vi "InitializeAll.vi"(8 "Error In":errorcluster) -> (0 "Error Out":errorcluster, 3 "CommunicationRefs":T8)   [LabVIEW 2015]
uses:
  TypeDefs/CoriFlowSettings.ctl
  TypeDefs/CommunicationRefs.ctl
  TypeDefs/MessageCluster.ctl
  TypeDefs/MPXSettings.ctl
  TypeDefs/ClsSettings.ctl
  TypeDefs/PDCSettings.ctl
  TypeDefs/JW24F14Settings.ctl
  TypeDefs/DAQmxAcqSettings.ctl
panel:
  in  "READY":bool
  in  "Settings":T1(tab)=enum."Photron PDC"
  in  "DAQmxAcq Settings":T2={"DAQmx Channel"="", "Simulate"=TRUE}
  in  "CoriFlowSettings":T3={"FlowBUS COM-Port"="COM3", "Node"=3, "Baud Rate"=38400, "Control Mode (0: BUS/RS232)"=enum."BUS/RS232", "Simulate"=TRUE}
  in  "ClsSettings":T4={"Connection Info (IP)"="IP: 192.168.170.2", "Simulate"=TRUE, "Load Config?"=TRUE, "Path of CLS Config"=path "C:/ADP-SLA/Drop Impact Teststand/Config/CLS.xml", "Command "=""}
  in  "MPXSettings":T5={"MPX Port"="COM4", "Simulate"=TRUE}
  in  "PDCSettings":T6={"Interface"=enum."Gigabit-Ethernet", "AutoSearch"=TRUE, "IP - AutoSearch"=[192, 168, 0], "IP - Direct"=[192, 168, 0, 9], "Simulate"=TRUE}
  in  "JW24F14Settings":T7={"Simulate"=TRUE, "device index"=0}
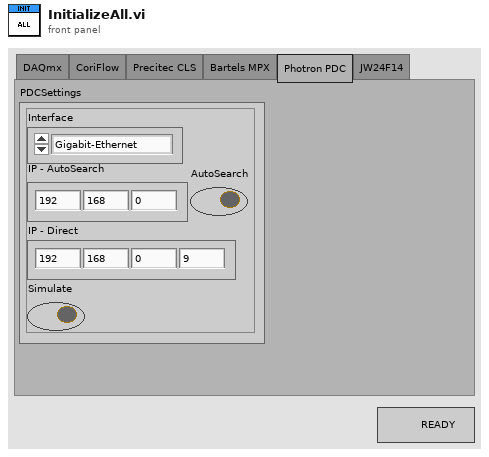
[diagram p1: front panel]
types:
  T1 = enum32{"DAQmx", "CoriFlow", "Precitec CLS", "Bartels MPX", "Photron PDC", "JW24F14"}
  T2 = typedef "DAQmxAcqSettings.ctl" = cluster{"DAQmx Channel":tag, "Simulate":bool}
  T3 = typedef "CoriFlowSettings.ctl" = cluster{"FlowBUS COM-Port":refnum<visa-resource-name>, "Node":u8, "Baud Rate":u32, "Control Mode (0: BUS/RS232)":enum32{"BUS/RS232", "Analog input", "FLOW-BUS slave", "Valve close", "Controller idle", "Testing mode", "Tuning mode", "Setpoint 100%", "Valve fully open", "Calibration mode", "Analog slave", "Keyboard or FLOW-BUS setpoint", "Setpoint 0%", "FLOW-BUS analog slave", "(FPP) Range select mode", "(FPP) Manual start sensor select, automatic end sensor", "(FPP) Automatic start sensor select, manual end sensor", "(FPP) Automatic start and end sensor", "RS232 Setpoint", "RS232 broadcast mode", "Valve stearing (valve = setpoint)", "Analog valve stearing (valve = analog setpoint)", "Valve safe state"}, "Simulate":bool}
  T4 = typedef "ClsSettings.ctl" = cluster{"Connection Info (IP)":string, "Simulate":bool, "Load Config?":bool, "Path of CLS Config":path, "Command ":string}
  T5 = typedef "MPXSettings.ctl" = cluster{"MPX Port":refnum<visa-resource-name>, "Simulate":bool}
  T6 = typedef "PDCSettings.ctl" = cluster{"Interface":enum16{"Gigabit-Ethernet", "IEEE1394a", "Photron Optical", "PCI/PCI Express"}, "AutoSearch":bool, "IP - AutoSearch":u32[], "IP - Direct":u32[], "Simulate":bool}
  T7 = typedef "JW24F14Settings.ctl" = cluster{"Simulate":bool, "device index":i32}
  T8 = typedef "CommunicationRefs.ctl" = cluster{"ErrorEvent":refnum<user-event>, "DataDisplay":refnum<queue>, "DAQmxAcq":refnum<queue>, "CoriFlow":refnum<queue>, "PrecitecCLS":refnum<queue>, "BartelsMPX":refnum<queue>, "PhotronPDC":refnum<queue>, "JW24F14":refnum<queue>, "Regulator":refnum<queue>, "Logging":refnum<queue>}
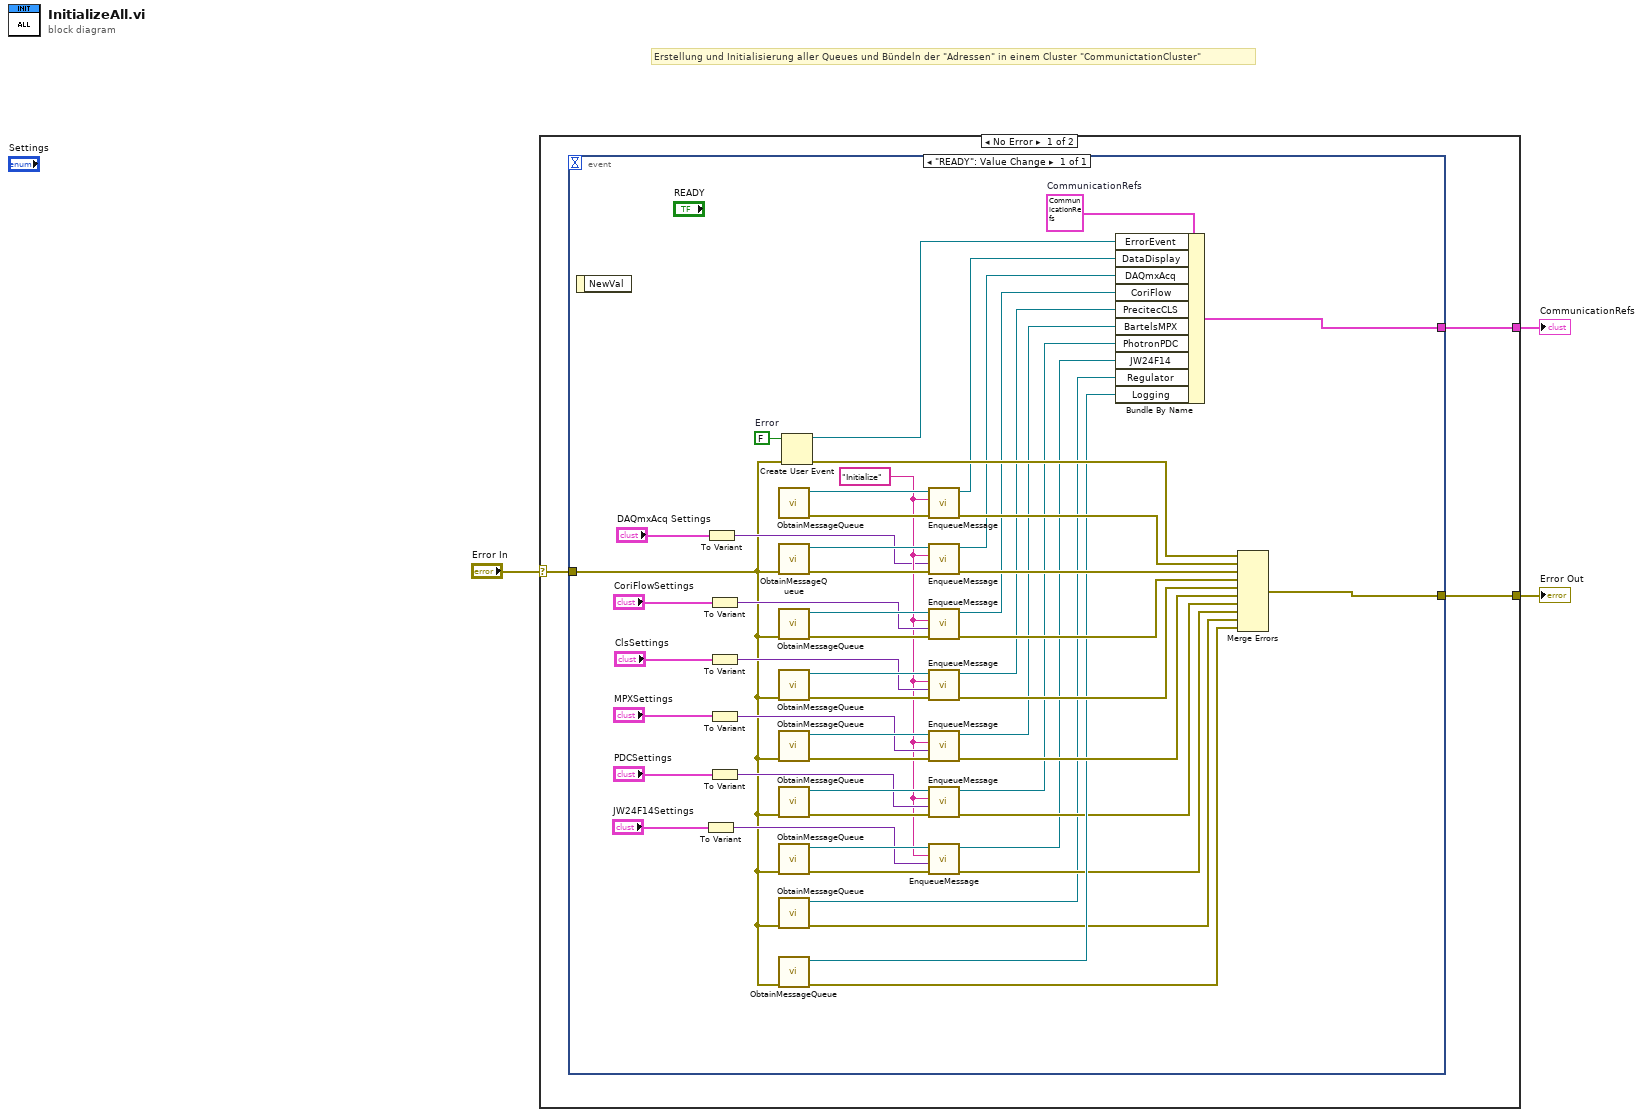
[diagram p0: block diagram]
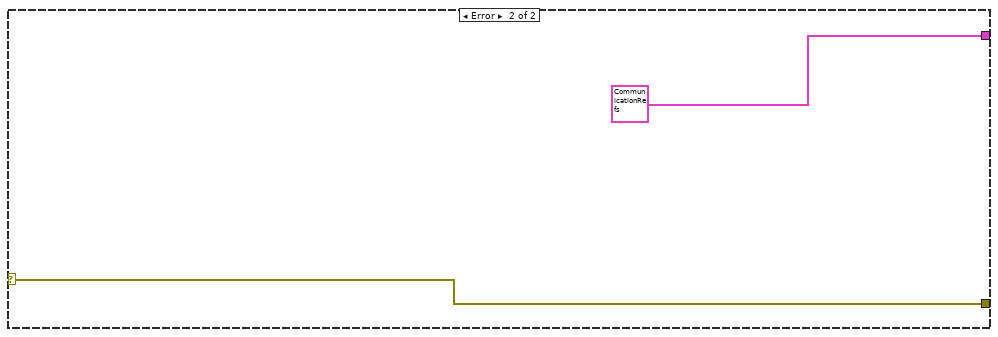
[diagram p2: hidden frame]
diagram:
  # "Erstellung und Initialisierung aller Queues und Bündeln der \"Adressen\" in einem Cluster \"CommunictationCluster\""
  n1 = case shown="No Error" "Error In" {
    selector: "Error In" -> [w4 w60]
    tunnel: [w5 w60] -> w2
    tunnel: [w6 T8 {"ErrorEvent"=refnum, "DataDisplay"=refnum, "DAQmxAcq"=refnum, "CoriFlow"=refnum, "PrecitecCLS"=refnum, "BartelsMPX"=refnum, "PhotronPDC"=refnum, "JW24F14"=refnum, "Regulator"=refnum, "Logging"=refnum} ("CommunicationRefs")] -> w1
    frame No Error {
      n2 = event shown="[0] \"READY\": Value Change" {
        selector: _ -> [_]
        dyn-events: _ -> [_]
        timeout: _ -> [_]
        tunnel: [w33] -> w6
        tunnel: [w32] -> w5
        tunnel: w4 -> [w7]
        event "READY": Value Change {
          w39 = FALSE  # Error
          w50 = T8 {"ErrorEvent"=refnum, "DataDisplay"=refnum, "DAQmxAcq"=refnum, "CoriFlow"=refnum, "PrecitecCLS"=refnum, "BartelsMPX"=refnum, "PhotronPDC"=refnum, "JW24F14"=refnum, "Regulator"=refnum, "Logging"=refnum}  # CommunicationRefs
          w15 = "Initialize" ("Message")
          n3 = event-data() -> ()  [unwired: 1 in, 1 out]
          n4 = To Variant(anything="JW24F14Settings") -> (Variant=w13:variant)
          n5 = To Variant(anything="DAQmxAcq Settings") -> (Variant=w11:variant)
          n6 = To Variant(anything="CoriFlowSettings") -> (Variant=w30:variant)
          n7 = To Variant(anything="ClsSettings") -> (Variant=w29:variant)
          n8 = To Variant(anything="MPXSettings") -> (Variant=w28:variant)
          n9 = To Variant(anything="PDCSettings") -> (Variant=w20:variant)
          n10 = call "ObtainMessageQueue.vi"() -> ("error out"=w36:errorcluster, "MessageQueue"=w37:refnum<queue>)  [unwired: 10 in]
          n11 = call "ObtainMessageQueue.vi"("error in (no error)"=w7) -> ("error out"=w53:errorcluster, "MessageQueue"=w52:refnum<queue>)  [unwired: 9 in]
          n12 = call "ObtainMessageQueue.vi"("error in (no error)"=w7) -> ("error out"=w47:errorcluster, "MessageQueue"=w48:refnum<queue>)  [unwired: 9 in]
          n13 = call "ObtainMessageQueue.vi"("error in (no error)"=w7) -> ("error out"=w45:errorcluster, "MessageQueue"=w44:refnum<queue>)  [unwired: 9 in]
          n14 = call "ObtainMessageQueue.vi"("error in (no error)"=w7) -> ("error out"=w42:errorcluster, "MessageQueue"=w43:refnum<queue>)  [unwired: 9 in]
          n15 = call "ObtainMessageQueue.vi"("error in (no error)"=w7) -> ("error out"=w25:errorcluster, "MessageQueue"=w23:refnum<queue>)  [unwired: 9 in]
          n16 = call "ObtainMessageQueue.vi"("error in (no error)"=w7) -> ("error out"=w18:errorcluster, "MessageQueue"=w19:refnum<queue>)  [unwired: 9 in]
          n17 = call "ObtainMessageQueue.vi"("error in (no error)"=w7) -> ("error out"=w9:errorcluster, "MessageQueue"=w10:refnum<queue>)  [unwired: 9 in]
          n18 = call "ObtainMessageQueue.vi"("error in (no error)"=w7) -> ("error out"=w8:errorcluster, "MessageQueue"=w34:refnum<queue>)  [unwired: 9 in]
          n19 = Create User Event(user event datatype=w39, error in=w7) -> (user event=w38:refnum<user-event>, error out=w57:errorcluster)
          n20 = call "EnqueueMessage.vi"("error in (no error)"=w36, "Message"=w15, "MessageQueue"=w37) -> ("error out"=w58:errorcluster, "dupMessageQueue"=w35:refnum<queue>)  [unwired: 7 in]
          n21 = call "EnqueueMessage.vi"("error in (no error)"=w53, "MessageData"=w11, "Message"=w15, "MessageQueue"=w52) -> ("error out"=w51:errorcluster, "dupMessageQueue"=w49:refnum<queue>)  [unwired: 6 in]
          n22 = call "EnqueueMessage.vi"("error in (no error)"=w47, "MessageData"=w30, "Message"=w15, "MessageQueue"=w48) -> ("error out"=w56:errorcluster, "dupMessageQueue"=w46:refnum<queue>)  [unwired: 6 in]
          n23 = call "EnqueueMessage.vi"("error in (no error)"=w45, "MessageData"=w29, "Message"=w15, "MessageQueue"=w44) -> ("error out"=w55:errorcluster, "dupMessageQueue"=w41:refnum<queue>)  [unwired: 6 in]
          n24 = call "EnqueueMessage.vi"("error in (no error)"=w42, "MessageData"=w28, "Message"=w15, "MessageQueue"=w43) -> ("error out"=w54:errorcluster, "dupMessageQueue"=w40:refnum<queue>)  [unwired: 6 in]
          n25 = call "EnqueueMessage.vi"("error in (no error)"=w25, "MessageData"=w20, "Message"=w15, "MessageQueue"=w23) -> ("error out"=w24:errorcluster, "dupMessageQueue"=w22:refnum<queue>)  [unwired: 6 in]
          n26 = call "EnqueueMessage.vi"("error in (no error)"=w18, "MessageData"=w13, "Message"=w15, "MessageQueue"=w19) -> ("error out"=w16:errorcluster, "dupMessageQueue"=w17:refnum<queue>)  [unwired: 6 in]
          n27 = Bundle By Name(cluster=w50, "ErrorEvent"=w38, "DataDisplay"=w35, "DAQmxAcq"=w49, "CoriFlow"=w46, "PrecitecCLS"=w41, "BartelsMPX"=w40, "PhotronPDC"=w22, "JW24F14"=w17, "Regulator"=w10, "Logging"=w34) -> (w33:T8)
          n28 = Merge Errors(w57, w58, w51, w56, w55, w54, w24, w16, w9, w8) -> (w32:errorcluster)
        }
      }
    }
    frame Error {
    }
  }
  "Error Out" <- w2
  "CommunicationRefs" <- w1
